vi "DAQ_Stop.vi"(8 "error in (no error)":errorcluster, 11 "Inputs":T1={"File Name"="", "Force (Hz)"=0.0, "Camera (Hz)"=0.0, "Systole (V)"=0.0, "Diastole (V)"=0.0, "T (sec)"=0.0, "Delay (sec)"=0.0, "Setpoint Function"=enum."Incremental PWM Step", "Max Diam (mm)"=0.0, "DAQmx Servo Task"="MyPulseOutputTask", "Force Sensor Channel"="Dev2/ai7", "DAQmx LED Task"="MyDigitalOutTask", "Camera Selector"="cam5", "FS Task Out"="", "Servo Task Out"="", "LED Task Out"="", "Camera Session Out"="", "Color Pane"=0} {"Color Pane" items=["Blue", "Red", "Green", "Saturation", "Value", "Intensity", "Luminance", "Hue", ""]}) -> (0 "error out":errorcluster)   [LabVIEW 2020]
uses:
  Controls/Inputs.ctl
  Controls/Serpoint.ctl
  <vilib>/userDefined/High Color/IMAQdx.ctl
panel:
  # "Test Variables:"
  # "Sampling Frequencies:"
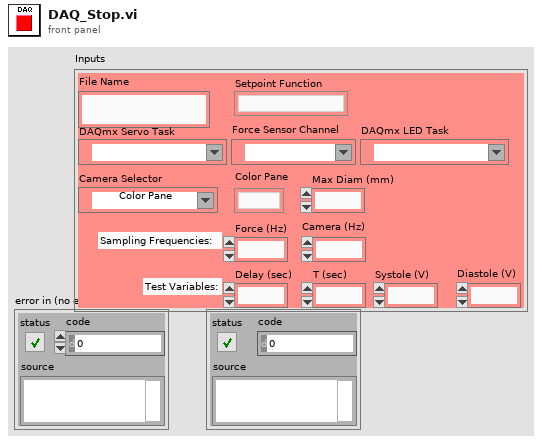
[diagram p1: front panel]
types:
  T1 = typedef "Inputs.ctl" = cluster{"File Name":string, "Force (Hz)":dbl, "Camera (Hz)":dbl, "Systole (V)":dbl, "Diastole (V)":dbl, "T (sec)":dbl, "Delay (sec)":dbl, "Setpoint Function":T2, "Max Diam (mm)":dbl, "DAQmx Servo Task":refnum<k21>, "Force Sensor Channel":tag, "DAQmx LED Task":refnum<k21>, "Camera Selector":T3, "FS Task Out":refnum<k21>, "Servo Task Out":refnum<k21>, "LED Task Out":refnum<k21>, "Camera Session Out":T3, "Color Pane":i32}
  T2 = typedef "Serpoint.ctl" = enum16{"Incremental PWM Step", "PWM Step", "Ramp", "Sinusoidal", "Blood-Pressure"}
  T3 = typedef "IMAQdx.ctl" = refnum<k21>
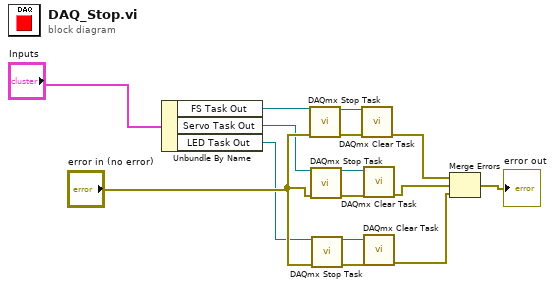
[diagram p0: block diagram]
diagram:
  n1 = Unbundle By Name("Inputs") -> ("FS Task Out"=w7:refnum<k21>, "Servo Task Out"=w8:refnum<k21>, "LED Task Out"=w9:refnum<k21>)
  n2 = call <vilib>:"DAQmx Stop Task.vi"("task/channels in"=w7, "error in"="error in (no error)") -> ("task out"=w5:refnum<k21>, "error out"=w6:errorcluster)  [unwired: 12 in]
  n3 = call <vilib>:"DAQmx Stop Task.vi"("task/channels in"=w8, "error in"="error in (no error)") -> ("task out"=w2:refnum<k21>, "error out"=w3:errorcluster)  [unwired: 12 in]
  n4 = call <vilib>:"DAQmx Stop Task.vi"("task/channels in"=w9, "error in"="error in (no error)") -> ("task out"=w4:refnum<k21>, "error out"=w11:errorcluster)  [unwired: 12 in]
  n5 = call <vilib>:"DAQmx Clear Task.vi"("task in"=w5, "error in"=w6) -> ("error out"=w12:errorcluster)  [unwired: 13 in]
  n6 = call <vilib>:"DAQmx Clear Task.vi"("task in"=w2, "error in"=w3) -> ("error out"=w13:errorcluster)  [unwired: 13 in]
  n7 = call <vilib>:"DAQmx Clear Task.vi"("task in"=w4, "error in"=w11) -> ("error out"=w14:errorcluster)  [unwired: 13 in]
  n8 = Merge Errors(w12, w13, w14) -> (→"error out":errorcluster)
